vi "Convert360.vi"(1 "Reverse":bool, 2 "Current Position":dbl, 3 "Zero Position":dbl) -> (0 "Angle":dbl)   [LabVIEW 2016]
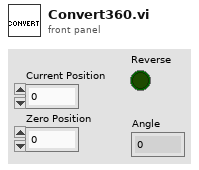
[diagram p1: front panel]
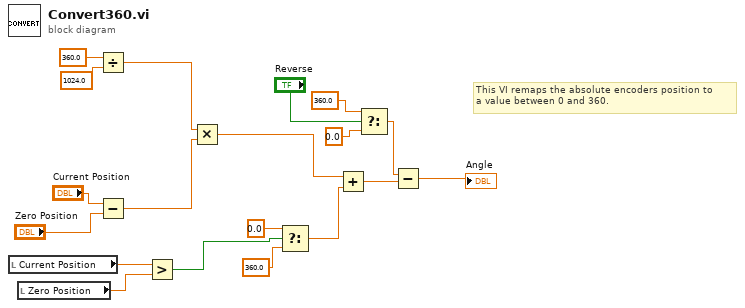
[diagram p0: block diagram]
diagram:
  # "This VI remaps the absolute encoders position to \na value between 0 and 360."
  n1 = local read "Current Position"() -> (w9:dbl)
  n2 = local read "Zero Position"() -> (w7:dbl)
  n3 = Divide(x=360.0, y=1024.0) -> (x/y=w19:dbl)
  n4 = Subtract(x="Current Position", y="Zero Position") -> (x-y=w18:dbl)
  n5 = Greater?(x=w9, y=w7) -> (0:w8:bool)
  n6 = Multiply(x=w19, y=w18) -> (x*y=w12:dbl)
  n7 = Select(t=0.0, s=w8, f=360.0) -> (s? t:f=w13:dbl)
  n8 = Add(x=w12, y=w13) -> (x+y=w6:dbl)
  n9 = Select(t=360.0 ("x"), s="Reverse", f=0.0 ("x")) -> (s? t:f=w4:dbl)
  n10 = Subtract(x=w4, y=w6) -> (x-y=→"Angle":dbl)
